vi "GetDelegateFunctionPointer.vi"(9 "target class":refnum<k24>, 10 "error in (no error)":errorcluster, 11 "event callback refnum":refnum<k27>) -> (0 "error out":errorcluster, 2 "(*f)(...)":i32, 3 "References":T1)   [LabVIEW 2011]
uses:
  C:/Users/Behavior Room/Desktop/Kinect Mouse/DepthSense/FunctionPointerProxy/FunctionPointerProxy/bin/Release/FunctionPointerProxy.dll
  FunctionPointerProxy/FunctionPointerProxy/bin/Release/FunctionPointerProxy.dll
  FunctionPointerProxy/LabVIEW/t_CallbackReferences.ctl
panel:
  # "//Copyright (c) 2006 Bruno van Dooren\n//Permission is hereby granted, free of charge, to any person obtaining a copy\n//of this software and associated documentation files (the \"Software\"), to deal\n//in the Software without restriction, including without limitation the rights\n//to use, copy, modify, merge, publish, distribute, sublicense, and/or sell\n//copies of the Software, and to permit persons to whom the Software is\n//furnished to do so, subject to the following conditions:\n//The above copyright notice and this permission notice shall be included in all\n//copies or substantial portions of the Software.\n//THE SOFTWARE IS PROVIDED \"AS IS\", WITHOUT WARRANTY OF ANY KIND, EXPRESS OR\n//IMPLIED, INCLUDING BUT NOT LIMITED TO THE WARRANTIES OF MERCHANTABILITY,\n//FITNESS FOR A PARTICULAR PURPOSE AND NONINFRINGEMENT. IN NO EVENT SHALL THE\n//AUTHORS OR COPYRIGHT HOLDERS BE LIABLE FOR ANY CLAIM, DAMAGES OR OTHER\n//LIABILITY, WHETHER IN AN ACTION OF CONTRACT, TORT OR OTHERWISE, ARISING FROM,\n//OUT OF OR IN CONNECTION WITH THE SOFTWARE OR THE USE OR OTHER DEALINGS IN THE\n//SOFTWARE."
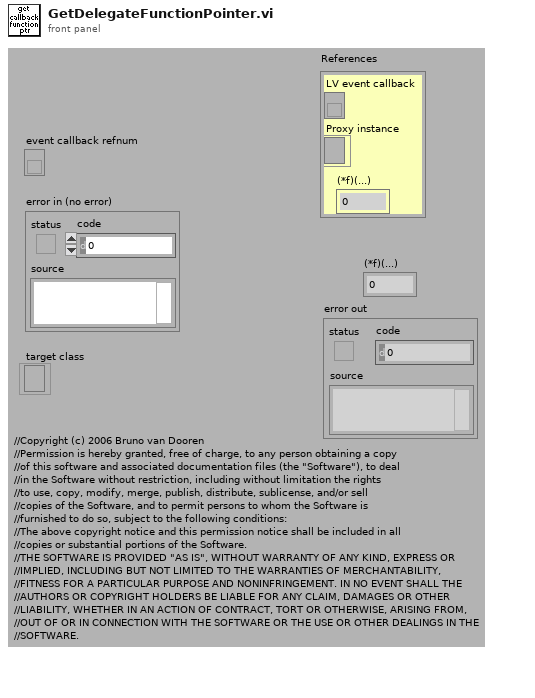
[diagram p1: front panel]
types:
  T1 = typedef "t_CallbackReferences.ctl" = cluster{"LV event callback ":refnum<k27>, "Proxy instance":refnum<k24>, "(*f)(...)":i32}
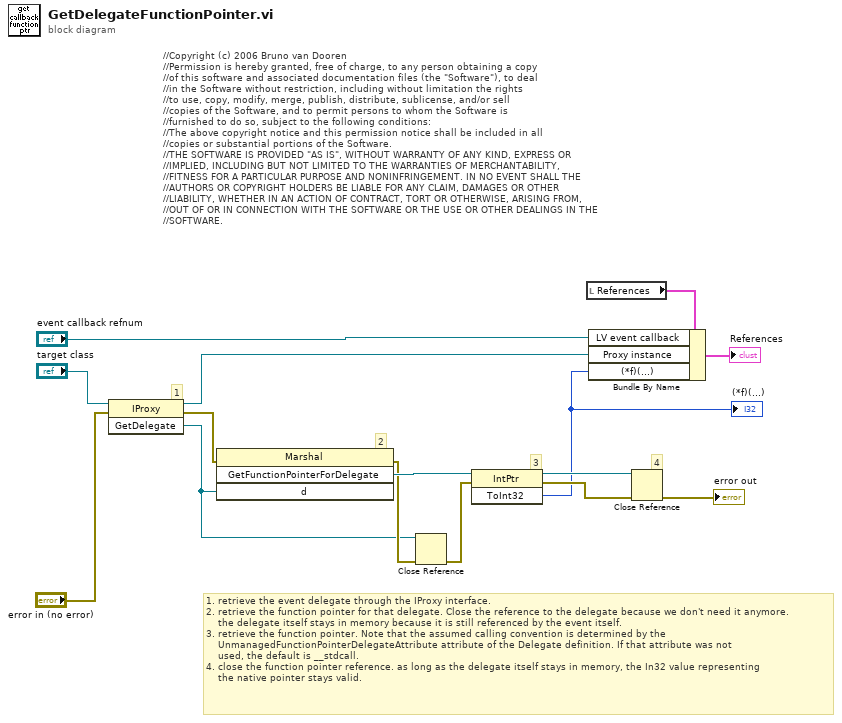
[diagram p0: block diagram]
diagram:
  # "//Copyright (c) 2006 Bruno van Dooren\n//Permission is hereby granted, free of charge, to any person obtaining a copy\n//of this software and associated documentation files (the \"Software\"), to deal\n//in the Software without restriction, including without limitation the rights\n//to use, copy, modify, merge, publish, distribute, sublicense, and/or sell\n//copies of the Software, and to permit persons to whom the Software is\n//furnished to do so, subject to the following conditions:\n//The above copyright notice and this permission notice shall be included in all\n//copies or substantial portions of the Software.\n//THE SOFTWARE IS PROVIDED \"AS IS\", WITHOUT WARRANTY OF ANY KIND, EXPRESS OR\n//IMPLIED, INCLUDING BUT NOT LIMITED TO THE WARRANTIES OF MERCHANTABILITY,\n//FITNESS FOR A PARTICULAR PURPOSE AND NONINFRINGEMENT. IN NO EVENT SHALL THE\n//AUTHORS OR COPYRIGHT HOLDERS BE LIABLE FOR ANY CLAIM, DAMAGES OR OTHER\n//LIABILITY, WHETHER IN AN ACTION OF CONTRACT, TORT OR OTHERWISE, ARISING FROM,\n//OUT OF OR IN CONNECTION WITH THE SOFTWARE OR THE USE OR OTHER DEALINGS IN THE\n//SOFTWARE."
  # "1. retrieve the event delegate through the IProxy interface.\n2. retrieve the function pointer for that delegate. Close the reference to the delegate because we don't need it anymore.\n    the delegate itself stays in memory because it is still referenced by the event itself.\n3. retrieve the function pointer. Note that the assumed calling convention is determined by the\n    UnmanagedFunctionPointerDelegateAttribute attribute of the Delegate definition. If that attribute was not\n    used, the default is __stdcall.\n4. close the function pointer reference. as long as the delegate itself stays in memory, the In32 value representing\n    the native pointer stays valid."
  # "4"
  # "3"
  # "2"
  # "1"
  n1 = invoke class="IProxy" method="GetDelegate"(reference="target class", error in="error in (no error)") -> (reference out=w8:refnum<k24>, error out=w14:errorcluster, "GetDelegate"=w6:refnum<k24>)  [unwired: 1 in]
  n2 = invoke class="Marshal" method="GetFunctionPointerForDelegate"(error in=w14, "d"=w6) -> (error out=w7:errorcluster, "GetFunctionPointerForDelegate"=w15:refnum<k24>)  [unwired: 2 in, 2 out]
  n3 = Close Reference(reference=w6, error in (no error)=w7) -> (error out=w5:errorcluster)
  n4 = invoke class="IntPtr" method="ToInt32"(reference=w15, error in=w5) -> (reference out=w13:refnum<k24>, error out=w12:errorcluster, "ToInt32"=w1:i32)  [unwired: 1 in]
  "(*f)(...)" <- w1
  n5 = local read "References"() -> (w10:T1)
  n6 = Bundle By Name(cluster=w10, "LV event callback"="event callback refnum", "Proxy instance"=w8, "(*f)(...)"=w1) -> (→"References":T1)
  n7 = Close Reference(reference=w13, error in (no error)=w12) -> (error out=→"error out":errorcluster)
